vi "send_data.vi"(2 "header size":i8=10, 3 "error in":errorcluster, 4 "Cluster":cluster{"type":string, "content":string}={"type"="hello", "content"="hello again"}, 5 "connection ID":refnum<k5>) -> (0 "error out":errorcluster, 1 "connection ID out":refnum<k5>)   [LabVIEW 2018]
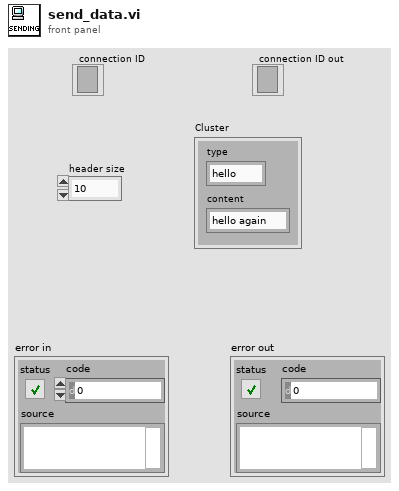
[diagram p1: front panel]
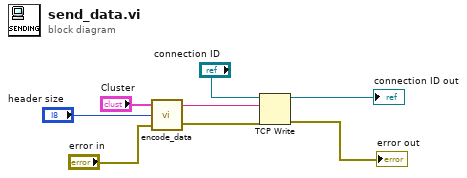
[diagram p0: block diagram]
diagram:
  n1 = call "encode_data.vi"("error in"="error in", "header size"="header size", "Cluster"="Cluster") -> ("error out"=w3:errorcluster, "encode_string"=w6:string)
  n2 = TCP Write(connection ID="connection ID", data in=w6, error in (no error)=w3) -> (connection ID out=→"connection ID out":refnum<k5>, error out=→"error out":errorcluster)  [unwired: 1 in, 1 out]
